vi "HFRR ADV v01.vi"() -> ()   [LabVIEW 2025] (continued)
                }
                frame 27 {
                  n3474 = property on="Boolean  4" class="Bool (strict)"("Boolean Text.Text"=w4454) -> ()  [unwired: 2 in, 2 out]
                }
                frame 28 {
                  n3475 = property on="Test \nStatus" class="Bool (strict)"("Boolean Text.Text"=w4455) -> ()  [unwired: 2 in, 2 out]
                }
                frame 29 {
                }
                frame 30 {
                }
                frame 31 {
                }
                frame 32 {
                  n3476 = property on="RSTCOF" class="Bool"("Boolean Text.Text"=w4457) -> ()  [unwired: 2 in, 2 out]
                  n3477 = property on="RST FF" class="Bool"("Boolean Text.Text"=w4457) -> ()  [unwired: 2 in, 2 out]
                  n3478 = property on="RST TEMP" class="Bool"("Boolean Text.Text"=w4457) -> ()  [unwired: 2 in, 2 out]
                  n3479 = property on="RSTV1 3" class="Bool"("Boolean Text.Text"=w4457) -> ()  [unwired: 2 in, 2 out]
                  n3480 = property on="rstv2" class="Bool"("Boolean Text.Text"=w4457) -> ()  [unwired: 2 in, 2 out]
                  n3481 = property on="RSTV1 2" class="Bool"("Boolean Text.Text"=w4457) -> ()  [unwired: 2 in, 2 out]
                  n3482 = property on="RST CP" class="Bool"("Boolean Text.Text"=w4457) -> ()  [unwired: 2 in, 2 out]
                }
                frame 33 {
                  "S 61" <- w4458
                }
                frame 34 {
                  "String 23" <- w4459
                }
                frame 35 {
                  n3483 = property on="Rh Before" class="DigNum (strict)"("Caption.Text"=w4460) -> ()  [unwired: 2 in, 2 out]
                }
                frame 36 {
                  n3484 = Match Pattern(string=w4461, regular expression=",") -> (before substring=→"bs":string, after substring=→"as":string)  [unwired: 1 in, 2 out]
                  n3485 = property on="Rh After" class="DigNum (strict)"("Caption.Text"=w4461) -> ()  [unwired: 2 in, 2 out]
                }
                frame 37 {
                  n3486 = Match Pattern(string=w4470, regular expression=",") -> (before substring=w4469:string, after substring=w4468:string)  [unwired: 1 in, 2 out]
                  "bs" <- w4469
                  "as" <- w4468
                  n3487 = Concatenate Strings(w4469, w4468) -> (w4465:string)
                  n3488 = property on="Humidity before test 2" class="DigNum (strict)"("Caption.Text"=w4465) -> ()  [unwired: 2 in, 2 out]
                  n3489 = Concatenate Strings(w4465, "=" ("string")) -> (w4466:string)
                  n3490 = local write "S 38"(w4466) -> ()
                }
                frame 38 {
                  n3491 = Match Pattern(string=w4477, regular expression=",") -> (before substring=w4476:string, after substring=w4475:string)  [unwired: 1 in, 2 out]
                  "bs" <- w4476
                  "as" <- w4475
                  n3492 = Concatenate Strings(w4476, w4475) -> (w4472:string)
                  n3493 = property on="Humidity after test 2" class="DigNum (strict)"("Caption.Text"=w4472) -> ()  [unwired: 2 in, 2 out]
                  n3494 = Concatenate Strings(w4472, "=" ("string")) -> (w4474:string)
                  n3495 = local write "S 39"(w4474) -> ()
                }
                frame 39 {
                  n3496 = Match Pattern(string=w4484, regular expression=",") -> (before substring=w4483:string, after substring=w4482:string)  [unwired: 1 in, 2 out]
                  "bs" <- w4483
                  "as" <- w4482
                  n3497 = Concatenate Strings(w4483, w4482) -> (w4479:string)
                  n3498 = property on="Temperature before test 2" class="DigNum (strict)"("Caption.Text"=w4479) -> ()  [unwired: 2 in, 2 out]
                  n3499 = Concatenate Strings(w4479, "=" ("string")) -> (→"String 34":string)
                }
                frame 40 {
                  n3500 = Match Pattern(string=w4491, regular expression=",") -> (before substring=w4490:string, after substring=w4489:string)  [unwired: 1 in, 2 out]
                  "bs" <- w4490
                  "as" <- w4489
                  n3501 = Concatenate Strings(w4490, w4489) -> (w4486:string)
                  n3502 = property on="Temperature after test 2" class="DigNum (strict)"("Caption.Text"=w4486) -> ()  [unwired: 2 in, 2 out]
                  n3503 = Concatenate Strings(w4486, "=" ("string")) -> (→"String 35":string)
                  n3504 = property on="Temperature after test" class="DigNum (strict)"("Caption.Text"=w4486) -> ()  [unwired: 2 in, 2 out]
                }
                frame 41 {
                  n3505 = property on="AVP 2" class="DigNum (strict)"("Caption.Text"=w4495) -> ()  [unwired: 2 in, 2 out]
                  n3506 = Concatenate Strings(w4495, "=" ("string")) -> (→"String 36":string)
                }
                frame 42 {
                  n3507 = property on="MWSD 2" class="DigNum (strict)"("Caption.Text"=w4498) -> ()  [unwired: 2 in, 2 out]
                  n3508 = Concatenate Strings(w4498, "=" ("string")) -> (→"String 37":string)
                }
                frame 43 {
                  n3509 = property on="HCF 2" class="DigNum (strict)"("Caption.Text"=w4501) -> ()  [unwired: 2 in, 2 out]
                  n3510 = Concatenate Strings(w4501, "=" ("string")) -> (→"String 38":string)
                }
                frame 44 {
                  n3511 = Concatenate Strings(w4503, "=" ("string")) -> (→"String 39":string)
                  n3512 = property on="WS1.4 2" class="DigNum (strict)"("Caption.Text"=w4503) -> ()  [unwired: 2 in, 2 out]
                }
                frame 45 {
                }
                frame 46 {
                  n3513 = local write "S 47"(w4506) -> ()
                }
                frame 47 {
                  n3514 = local write "S 48"(w4507) -> ()
                }
                frame 48 {
                  n3515 = local write "S 49"(w4508) -> ()
                }
                frame 49 {
                  n3516 = local write "S 50"(w4509) -> ()
                }
                frame 50 {
                  n3517 = local write "S 51"(w4510) -> ()
                }
                frame 51 {
                  n3518 = local write "S 52"(w4511) -> ()
                }
                frame 52 {
                  n3519 = local write "S 53"(w4512) -> ()
                }
                frame 53 {
                  n3520 = local write "S 54"(w4513) -> ()
                }
                frame 54 {
                  n3521 = local write "S 55"(w4514) -> ()
                }
                frame 55 {
                  n3522 = local write "S 56"(w4515) -> ()
                }
                frame 56 {
                  n3523 = local write "S 57"(w4516) -> ()
                }
                frame 57 {
                  n3524 = local write "S 58"(w4517) -> ()
                }
                frame 58 {
                  n3525 = local write "S 59"(w4518) -> ()
                }
                frame 59 {
                  n3526 = local write "S 60"(w4519) -> ()
                }
                frame 60 {
                  n3527 = local write "S 62"(w4520) -> ()
                }
                frame 61 {
                  n3528 = local write "S 63"(w4521) -> ()
                }
                frame 62 {
                  n3529 = local write "S 64"(w4522) -> ()
                }
                frame 63 {
                  n3530 = local write "S 65"(w4523) -> ()
                }
                frame 64 {
                  n3531 = local write "S 66"(w4524) -> ()
                }
                frame 65 {
                  n3532 = local write "S 67"(w4525) -> ()
                }
                frame 66 {
                  n3533 = local write "S 68"(w4526) -> ()
                }
                frame 67 {
                  n3534 = local write "S 69"(w4527) -> ()
                }
                frame 68 {
                  n3535 = local write "S 70"(w4528) -> ()
                }
                frame 69 {
                  n3536 = local write "S 71"(w4529) -> ()
                }
                frame 70 {
                  n3537 = local write "S 72"(w4530) -> ()
                }
                frame 71 {
                  n3538 = local write "S 73"(w4531) -> ()
                }
                frame 72 {
                  n3539 = local write "S 74"(w4532) -> ()
                }
                frame 73 {
                  n3540 = local write "S 75"(w4533) -> ()
                }
                frame 74 {
                  n3541 = local write "S 76"(w4534) -> ()
                }
                frame 75 {
                  n3542 = local write "S 77"(w4535) -> ()
                }
                frame 76 {
                  n3543 = local write "S 78"(w4536) -> ()
                }
                frame 77 {
                  n3544 = local write "S 79"(w4537) -> ()
                }
                frame 79 {
                  n3545 = property on="Sample Temperature ( °C )" class="XYGraph (strict)"("Y Scale.Name Label.Text"=w4538) -> ()  [unwired: 2 in, 2 out]
                }
                frame 80 {
                  n3546 = local write "S 81"(w4539) -> ()
                  n3547 = property on="Humidity ( %RH )" class="XYGraph (strict)"("Y Scale.Name Label.Text"=w4539) -> ()  [unwired: 2 in, 2 out]
                }
                frame 78 {
                  n3548 = property on="Air Temperature  ( °C )" class="XYGraph (strict)"("X Scale.Name Label.Text"=w4540) -> ()  [unwired: 2 in, 2 out]
                  n3549 = property on="Humidity ( %RH )" class="XYGraph (strict)"("X Scale.Name Label.Text"=w4540) -> ()  [unwired: 2 in, 2 out]
                  n3550 = property on="Sample Temperature ( °C )" class="XYGraph (strict)"("X Scale.Name Label.Text"=w4540) -> ()  [unwired: 2 in, 2 out]
                  n3551 = property on="Coefficient Of Friction" class="XYGraph (strict)"("X Scale.Name Label.Text"=w4540) -> ()  [unwired: 2 in, 2 out]
                }
                frame 81 {
                  n3552 = property on="Air Temperature  ( °C )" class="XYGraph (strict)"("Y Scale.Name Label.Text"=w4541) -> ()  [unwired: 2 in, 2 out]
                }
                frame 82 {
                  n3553 = local write "S 84"(w4542) -> ()
                }
                frame 83 {
                  n3554 = local write "S 85"(w4543) -> ()
                }
                frame 84 {
                  n3555 = local write "S 86"(w4544) -> ()
                }
                frame 85 {
                  n3556 = local write "S 87"(w4545) -> ()
                }
                frame 86 {
                  n3557 = local write "S 88"(w4546) -> ()
                }
                frame 87 {
                }
                frame 88 {
                  n3558 = local write "S 90"(w4548) -> ()
                }
                frame 89 {
                  n3559 = local write "S 91"(w4549) -> ()
                }
                frame 90 {
                  n3560 = local write "S 92"(w4550) -> ()
                }
                frame 91 {
                  n3561 = local write "S 93"(w4551) -> ()
                }
                frame 92 {
                  n3562 = local write "S 94"(w4552) -> ()
                }
                frame 93 {
                  n3563 = local write "S 95"(w4553) -> ()
                }
                frame 94 {
                  n3564 = local write "S 96"(w4554) -> ()
                }
                frame 95 {
                  n3565 = local write "S 97"(w4555) -> ()
                }
                frame 96 {
                  n3566 = local write "S 98"(w4556) -> ()
                }
                frame 97 {
                  n3567 = local write "S 99"(w4557) -> ()
                }
                frame 98 {
                  n3568 = local write "S 100"(w4558) -> ()
                }
                frame 99 {
                  n3569 = local write "S 101"(w4559) -> ()
                }
                frame 100 {
                  n3570 = local write "S 102"(w4560) -> ()
                }
                frame 101 {
                  n3571 = local write "S 103"(w4561) -> ()
                }
                frame 102 {
                  n3572 = local write "S 104"(w4562) -> ()
                }
                frame 103 {
                  n3573 = local write "S 105"(w4563) -> ()
                }
                frame 104 {
                  n3574 = local write "S 106"(w4564) -> ()
                }
                frame 105 {
                }
                frame 106 {
                  n3575 = property on="OK Button 17" class="Bool (strict)"("Boolean Text.Text"=w4565) -> ()  [unwired: 2 in, 2 out]
                }
                frame 107 {
                  n3576 = property on="OK Button 16" class="Bool (strict)"("Boolean Text.Text"=w4566) -> ()  [unwired: 2 in, 2 out]
                }
                frame 108 {
                  n3577 = property on="TITTLE" class="Str"("Caption.Text"=w4567) -> ()  [unwired: 2 in, 2 out]
                }
                frame 109 {
                  "String 30" <- w4568
                }
                frame 110 {
                  n3578 = property on="Test Date" class="Str"("Caption.Text"=w4569) -> ()  [unwired: 2 in, 2 out]
                  "String 31" <- w4569
                }
                frame 111 {
                  n3579 = property on="Sample ID" class="Str"("Caption.Text"=w4570) -> ()  [unwired: 2 in, 2 out]
                  "String 32" <- w4570
                }
                frame 112 {
                  n3580 = property on="Tested by" class="Str"("Caption.Text"=w4571) -> ()  [unwired: 2 in, 2 out]
                  "String 33" <- w4571
                }
                frame 113 {
                  n3581 = property on="System Configured Printers 2" class="Arr (strict)"("Caption.Text"=w4572) -> ()  [unwired: 2 in, 2 out]
                }
                frame 114 {
                  n3582 = property on="Selected Printer" class="Str"("Caption.Text"=w4573) -> ()  [unwired: 2 in, 2 out]
                }
                frame 115 {
                  n3583 = property on="Select Printer 3" class="DigNum (strict)"("Caption.Text"=w4574) -> ()  [unwired: 2 in, 2 out]
                }
                frame 116 {
                  n3584 = property on="Print" class="Bool (strict)"("Boolean Text.Text"=w4575) -> ()  [unwired: 2 in, 2 out]
                }
                frame 117 {
                  "String 41" <- w4576
                }
                frame 118 {
                  n3585 = property on="tested by" class="Str"("Caption.Text"=w4577) -> ()  [unwired: 2 in, 2 out]
                }
                frame 119 {
                }
                frame 120 {
                  n3586 = property on="Export" class="Bool (strict)"("Boolean Text.Text"=w4578) -> ()  [unwired: 2 in, 2 out]
                }
                frame 121 {
                }
                frame 122 {
                }
                frame 123 {
                  n3587 = property on="Select File Type" class="Enum (strict)"("Caption.Text"=w4581) -> ()  [unwired: 2 in, 2 out]
                }
                frame 124 {
                  n3588 = property on="s.NO" class="Str"("Caption.Text"=w4582) -> ()  [unwired: 2 in, 2 out]
                  "String 45" <- w4582
                }
                frame 125 {
                  n3589 = property on="trip1 8" class="Bool (strict)"("Boolean Text.Text"=w4583) -> ()  [unwired: 2 in, 2 out]
                }
                frame 126, Default {
                }
              }
            }
          }
          frame #1 {
            w4591 = TRUE ("Visible")
            n3590 = local read "S 91"() -> (w4608:string)
            n3591 = local read "S 90"() -> (w4607:string)
            n3592 = local read "S 88"() -> (w4606:string)
            n3593 = property on="File Path" class="Path"("Caption.Text"=w4607) -> ()  [unwired: 2 in, 2 out]
            n3594 = local read "S 71"() -> (w4601:string)
            n3595 = local read "S 86"() -> (w4603:string)
            n3596 = local read "S 85"() -> (w4604:string)
            n3597 = local read "S 87"() -> (w4602:string)
            n3598 = local read "S 84"() -> (w4605:string)
            n3599 = local read "S 103"() -> (w4590:string)
            n3600 = local read "S 104"() -> (w4589:string)
            n3601 = property on="Password" class="Str"("Caption.Text"=w4604) -> ()  [unwired: 2 in, 2 out]
            n3602 = property on="EDIT" class="Bool (strict)"("Boolean Text.Text"=w4601) -> ()  [unwired: 2 in, 2 out]
            n3603 = property on="SAVE" class="Bool (strict)"("Boolean Text.Text"=w4605) -> ()  [unwired: 2 in, 2 out]
            n3604 = Build Array(w4590, w4589) -> (w4588:string[])
            n3605 = property on="Heater Button" class="Bool (strict)"("Strings [4]"=w4588) -> ()  [unwired: 2 in, 2 out]
            n3606 = local read "S 92"() -> (w4600:string)
            n3607 = local read "S 93"() -> (w4599:string)
            n3608 = local read "S 105"() -> (w4586:string)
            n3609 = local read "S 106"() -> (w4585:string)
            n3610 = Build Array(w4600, w4599) -> ()  [unwired: 1 out]
            n3611 = Build Array(w4586, w4585) -> (w4587:string[])
            n3612 = local read "S 95"() -> (w4597:string)
            n3613 = local read "S 94"() -> (w4598:string)
            n3614 = local read "bs"() -> (w4613:string)
            n3615 = local read "as"() -> (w4614:string)
            n3616 = property on="Humidity" class="Bool (strict)"("Strings [4]"=w4587) -> ()  [unwired: 2 in, 2 out]
            n3617 = Concatenate Strings(w4613, "\r", w4614) -> ()  [unwired: 1 out]
            n3618 = property on="Rh After" class="DigNum (strict)"("Caption.Size to Text?"=TRUE ("Caption.Size to Text")) -> ()  [unwired: 2 in, 2 out]
            n3619 = local read "S 48"() -> (w4637:string)
            n3620 = local read "S 50"() -> (w4635:string)
            n3621 = local read "S 51"() -> (w4634:string)
            n3622 = local read "S 49"() -> (w4636:string)
            n3623 = local read "S 52"() -> (w4633:string)
            n3624 = local read "as"() -> (w4618:string)
            n3625 = local read "bs"() -> (w4619:string)
            n3626 = local read "S 56"() -> (w4632:string)
            n3627 = local read "S 57"() -> (w4631:string)
            n3628 = local read "S 58"() -> (w4630:string)
            n3629 = local read "S 59"() -> (w4629:string)
            n3630 = property on="OPEN" class="Bool (strict)"("Boolean Text.Text"=w4633) -> ()  [unwired: 2 in, 2 out]
            n3631 = property on="OPEN 1" class="Bool (strict)"("Boolean Text.Text"=w4637) -> ()  [unwired: 2 in, 2 out]
            n3632 = property on="OPEN 2" class="Bool (strict)"("Boolean Text.Text"=w4636) -> ()  [unwired: 2 in, 2 out]
            n3633 = property on="OPEN 3" class="Bool (strict)"("Boolean Text.Text"=w4635) -> ()  [unwired: 2 in, 2 out]
            n3634 = property on="OPEN 4" class="Bool (strict)"("Boolean Text.Text"=w4634) -> ()  [unwired: 2 in, 2 out]
            n3635 = Concatenate Strings(w4619, "\r", w4618) -> ()  [unwired: 1 out]
            n3636 = local read "S 102"() -> (w4592:string)
            n3637 = property on="КОФ1" class="DigNum (strict)"("Caption.Text"=w4632) -> ()  [unwired: 2 in, 2 out]
            n3638 = local read "S 98"() -> (w4596:string)
            n3639 = local read "S 99"() -> (w4595:string)
            n3640 = local read "S 100"() -> (w4594:string)
            n3641 = local read "S 101"() -> (w4593:string)
            n3642 = property on="КОФ2" class="DigNum (strict)"("Caption.Text"=w4631) -> ()  [unwired: 2 in, 2 out]
            n3643 = property on="КОФ3" class="DigNum (strict)"("Caption.Text"=w4630) -> ()  [unwired: 2 in, 2 out]
            n3644 = property on="КОФ4" class="DigNum (strict)"("Caption.Text"=w4629) -> ()  [unwired: 2 in, 2 out]
            n3645 = local read "bs"() -> (w4617:string)
            n3646 = local read "as"() -> (w4616:string)
            n3647 = local read "S 60"() -> (w4628:string)
            n3648 = local read "S 54"() -> (w4638:string)
            n3649 = Concatenate Strings(w4617, "\r", w4616) -> ()  [unwired: 1 out]
            n3650 = Concatenate Strings(w4638, w4628) -> ()  [unwired: 1 out]
            n3651 = local read "S 77"() -> (→"String 43":string)
            n3652 = local read "S 76"() -> (w4611:string)
            n3653 = local read "S 78"() -> (w4610:string)
            n3654 = local read "S 71"() -> (w4622:string)
            n3655 = local read "S 66"() -> (w4627:string)
            n3656 = local read "S 67"() -> (w4626:string)
            n3657 = local read "S 68"() -> (w4625:string)
            n3658 = local read "S 69"() -> (w4624:string)
            n3659 = local read "S 70"() -> (w4623:string)
            n3660 = property on="AIR TEMP" class="DigNum (strict)"("Caption.Text"=w4610) -> ()  [unwired: 2 in, 2 out]
            n3661 = property on="Set Strk" class="DigNum (strict)"("Caption.Text"=w4611) -> ()  [unwired: 2 in, 2 out]
            n3662 = property on="SPEED OUT:" class="DigNum (strict)"("Caption.Text"=w4625) -> ()  [unwired: 2 in, 2 out]
            n3663 = property on="EDIT" class="Bool (strict)"("Boolean Text.Text"=w4622) -> ()  [unwired: 2 in, 2 out]
            n3664 = local read "S 79"() -> (w4609:string)
          }
          frame #2 {
          }
        }
        n3665 = local write "Lan flag"(10.0 ("Lan flag")) -> ()
      }
      frame Enabled {
      }
    }
    n3666 = Wait (ms)(milliseconds to wait=u32 2000) -> ()  [unwired: 1 out]
    n3667 = local read "Quit"() -> (w4412:bool)
  }
  n3668 = while {
    shift-right: [w4644] -> _
    shift-left: _ -> [w4645]
    shift-right: [w4642] -> _
    shift-left: T19 {"Read Heave and Surge"="", "Bytes at Heave Port"=0.0, "Heave and Surge COM Port:"="COM9", "Com Port 2"="COM7", "Residual Due"="", "Heave COM Status 2"=TRUE, "Heave COM Status"=TRUE, "Port 2"=TRUE, "Sway PPR"=6400.0, "Surge PPR"=6400.0, "Heave PPR"=6400.0, "Sway Pitch"=2.0, "Surge Pitch"=3.0, "Heave Pitch"=4.0, "Sway Pulses/mm"=320.0, "Surge Pulses/mm"=1600.0, "Heave Pulses/mm"=1600.0, "inner loop"=0.0, "Read Heave and Surge 2"="", "String 36"="", "Write S"=FALSE, "WriteCC1"=[""], "Heave COM Loop"=0, "LastCom"="", "EXIT"=FALSE, "Error Heave"={"status"=TRUE, "code"=-1073807343, "source"=""}} -> [w4641]
    shift-right: [w4639] -> _
    shift-left: enum16{"init", "MAIN", "Panel Close"}."init" -> [w4640]
    stop <- w4643 stop-if-true
    # "HUMIDITY LOOP LOGIC"
    n3669 = case shown="\"MAIN\"" w4640 {
      tunnel: w4645 -> [w4659 w4684 w4783 w4785]
      tunnel: [w4654 w4668 w4783 w4785] -> w4644
      tunnel: [_ _ TRUE _] -> w4643
      tunnel: [w4651 w4669 w4781 w4784] -> w4642
      tunnel: w4641 -> [w4656 w4683 w4781 w4784]
      tunnel: [enum16{"init", "MAIN", "Panel Close"}."MAIN" w4678 _ _] -> w4639
      frame "init" {
        n3670 = local read "C3 :"() -> (w4646:refnum<visa-resource-name>)
        n3671 = Bundle By Name(cluster=w4656, "Heave and Surge COM Port:"=w4646) -> (w4655:T19)
        n3672 = call "Instrument fgv uno.vi"("Enum"=T32."INIT", "error in (no error) 2"=w4659, "INPUT"=w4655) -> ("error"=w4657:errorcluster, "output"=w4653:T19)  [unwired: 6 in, 1 out]
        n3673 = case shown="Error" w4657 {
          selector: w4657 -> [w4661 _]
          tunnel: [w4661 w4665] -> w4654
          tunnel: w4653 -> [w4660 w4663]
          tunnel: [w4660 w4662] -> w4652
          frame No Error {
          }
          frame Error {
            n3674 = call "Instrument fgv uno.vi"("Enum"=T32."ERROR INIT", "INPUT"=w4663) -> ("error"=w4666:errorcluster, "output"=w4662:T19)  [unwired: 7 in, 1 out]
            n3675 = call <vilib>:"Clear Errors.vi"("error in (no error)"=w4666) -> ("error out"=w4665:errorcluster)  [unwired: 5 in, 1 out]
          }
        }
        n3676 = local read "LastCom Humidity"() -> (w4649:string)
        n3677 = Unbundle By Name(w4652) -> ("Heave COM Status 2"=→"COM Status":bool, "Error Heave"=→"Error":errorcluster)  [unwired: 1 out]
        n3678 = Bundle By Name(cluster=w4652, "LastCom"=w4649) -> (w4651:T19)
      }
      frame "MAIN" {
        n3679 = Unbundle By Name(w4683) -> ("Com Port 2"=w4673:refnum<visa-resource-name>)
        n3680 = local read "C3 :"() -> (w4674:refnum<visa-resource-name>)
        n3681 = local write "COM Port Humidity :"(w4673) -> ()
        n3682 = Bundle By Name(cluster=w4683, "Heave and Surge COM Port:"=w4674) -> (w4682:T19)
        n3683 = Equal?(x=w4673, y=w4674) -> (x = y?=w4687:bool)
        n3684 = case shown="True" w4687 {
          tunnel: [w4727 w4745] -> w4672
          tunnel: w4684 -> [w4728 w4751]
          tunnel: w4682 -> [w4726 w4749]
          tunnel: [w4725 w4744] -> w4671
          frame False {
            n3685 = call <vilib>:"Clear Errors.vi"("error in (no error)"=w4728) -> ("error out"=w4724:errorcluster)  [unwired: 5 in, 1 out]
            n3686 = call "Instrument fgv uno.vi"("Enum"=T32."ERROR INIT", "error in (no error) 2"=w4724, "INPUT"=w4726) -> ("error"=w4730:errorcluster, "output"=w4725:T19)  [unwired: 6 in, 1 out]
            n3687 = call <vilib>:"Clear Errors.vi"("error in (no error)"=w4730) -> ("error out"=w4727:errorcluster)  [unwired: 5 in, 1 out]
          }
          frame True {
            n3688 = call "Instrument fgv uno.vi"("Enum"=T32."READ", "error in (no error) 2"=w4751, "milliseconds to wait"="milliseconds to wait 2", "INPUT"=w4749) -> ("error"=w4750:errorcluster, "output"=w4743:T19)  [unwired: 5 in, 1 out]
            n3689 = Bundle By Name(cluster=w4743, "String 36"="WRITE HUMIDITY") -> (w4742:T19)
            n3690 = case shown="True" "Write Humidity" {
              selector: "Write Humidity" -> [_ w4780]
              tunnel: w4750 -> [w4773 w4779]
              tunnel: [w4773 w4778] -> w4740
              tunnel: w4742 -> [w4772 w4776]
              tunnel: [w4772 w4775] -> w4739
              frame False {
              }
              frame True {
                n3691 = Not(x=w4780) -> (.not. x?=w4774:bool)
                n3692 = local write "Write Humidity"(w4774) -> ()
                n3693 = call "Instrument fgv uno.vi"("Enum"=T32."MANUAL WRITE", "error in (no error) 2"=w4779, "INPUT"=w4776) -> ("error"=w4778:errorcluster, "output"=w4775:T19)  [unwired: 6 in, 1 out]
              }
            }
            n3694 = Array Size(array="WriteHumidity") -> (size(s)=w4737:i32)
            n3695 = Greater Than 0?(x=w4737) -> (x > 0?=w4736:bool)
            n3696 = call "Instrument fgv uno.vi"("Enum"=T32."WRITE", "error in (no error) 2"=w4740, "WriteCC1"="WriteHumidity", "INPUT"=w4739) -> ("error"=w4747:errorcluster, "WriteCC1 2"=w4738:string[], "output"=w4746:T19)  [unwired: 5 in]
            n3697 = case shown="Error" w4747 {
              selector: w4747 -> [w4754 w4759]
              tunnel: w4746 -> [w4755 w4763]
              tunnel: [w4755 w4762] -> w4744
              tunnel: [w4754 w4760] -> w4745
              frame No Error {
              }
              frame Error {
                n3698 = Unbundle By Name(w4759) -> ("code"=w4758:i32)
                n3699 = Equal?(x=w4758, y=56) -> (x = y?=w4756:bool)
                n3700 = case shown="True" w4756 {
                  tunnel: w4763 -> [w4769 w4770]
                  tunnel: [w4768 w4770] -> w4762
                  tunnel: [w4767 w4771] -> w4761
                  tunnel: w4759 -> [w4764 w4771]
                  frame False {
                    n3701 = call <vilib>:"Clear Errors.vi"("error in (no error)"=w4764) -> ("error out"=w4765:errorcluster)  [unwired: 5 in, 1 out]
                    n3702 = call "Instrument fgv uno.vi"("Enum"=T32."ERROR INIT", "error in (no error) 2"=w4765, "INPUT"=w4769) -> ("error"=w4767:errorcluster, "output"=w4768:T19)  [unwired: 6 in, 1 out]
                  }
                  frame True {
                  }
                }
                n3703 = call <vilib>:"Clear Errors.vi"("error in (no error)"=w4761) -> ("error out"=w4760:errorcluster)  [unwired: 5 in, 1 out]
              }
            }
            n3704 = case shown="True" w4736 {
              tunnel: w4738 -> [_ w4753]
              frame False {
              }
              frame True {
                n3705 = local write "WriteHumidity"(w4753) -> ()
              }
            }
            n3706 = Unbundle By Name(w4744) -> ("LastCom"=→"LastCom Humidity":string, "Read Heave and Surge"=→"Read HUMIDITY":string)
          }
        }
        n3707 = Unbundle By Name(w4671) -> ("Heave COM Status 2"=w4686:bool, "Error Heave"=w4675:errorcluster, "Bytes at Heave Port"=→"Bytes at Humidity Port  2":dbl)  [unwired: 1 out]
        n3708 = Unbundle By Name(w4675) -> ("status"=→"Humidity Port":bool)
        n3709 = Not(x=w4686) -> (.not. x?=w4676:bool)
        n3710 = local write "Error"(w4675) -> ()
        n3711 = local read "Quit"() -> (w4679:bool)
        n3712 = local write "COM Status"(w4676) -> ()
        n3713 = Select(t=enum16{"init", "MAIN", "Panel Close"}."Panel Close", s=w4679, f=enum16{"init", "MAIN", "Panel Close"}."MAIN") -> (s? t:f=w4678:enum16{"init", "MAIN", "Panel Close"})
        n3714 = disable-structure shown="Enabled" {
          disable-tunnel: w4672 -> [w4692 w4704]
          disable-tunnel: w4671 -> [w4691 w4705]
          disable-tunnel: [w4689 w4705] -> w4670
          disable-tunnel: [w4688 w4704] -> w4667
          frame Disabled {
            n3715 = local read "Humidity 2"() -> (w4690:bool)
            n3716 = case shown="True" w4690 {
              selector: w4690 -> [_ w4695]
              tunnel: w4692 -> [w4693 w4700]
              tunnel: [w4693 w4699] -> w4688
              tunnel: w4691 -> [w4694 w4698]
              tunnel: [w4694 w4697] -> w4689
              frame False {
              }
              frame True {
                n3717 = Not(x=w4695) -> (.not. x?=→"Humidity 2":bool)
                n3718 = call <vilib>:"Clear Errors.vi"("error in (no error)"=w4700) -> ("error out"=w4703:errorcluster)  [unwired: 5 in, 1 out]
                n3719 = call "Instrument fgv uno.vi"("Enum"=T32."ERROR INIT", "error in (no error) 2"=w4703, "INPUT"=w4698) -> ("error"=w4701:errorcluster, "output"=w4697:T19)  [unwired: 6 in, 1 out]
                n3720 = call <vilib>:"Clear Errors.vi"("error in (no error)"=w4701) -> ("error out"=w4699:errorcluster)  [unwired: 5 in, 1 out]
              }
            }
          }
          frame Enabled {
          }
        }
        n3721 = case shown="Error .." w4667 {
          tunnel: w4670 -> [w4710 w4722]
          tunnel: w4667 -> [w4709 w4723]
          tunnel: [w4708 w4722] -> w4669
          tunnel: [w4707 w4723] -> w4668
          frame No Error {
            n3722 = First Call?() -> (First Call?: T/F=w4706:bool)
            n3723 = case shown="True" w4706 {
              tunnel: w4709 -> [w4711 w4718]
              tunnel: [w4711 w4717] -> w4707
              tunnel: w4710 -> [w4712 w4716]
              tunnel: [w4712 w4715] -> w4708
              frame False {
              }
              frame True {
                n3724 = call "Stall Data Flow.vim"("value in"=w4718, "milliseconds to wait"=u32 1000) -> ("value out"=w4714:errorcluster)  [unwired: 1 out]
                n3725 = call <vilib>:"Clear Errors.vi"("error in (no error)"=w4714) -> ("error out"=w4721:errorcluster)  [unwired: 5 in, 1 out]
                n3726 = call "Instrument fgv uno.vi"("Enum"=T32."ERROR INIT", "error in (no error) 2"=w4721, "INPUT"=w4716) -> ("error"=w4719:errorcluster, "output"=w4715:T19)  [unwired: 6 in, 1 out]
                n3727 = call <vilib>:"Clear Errors.vi"("error in (no error)"=w4719) -> ("error out"=w4717:errorcluster)  [unwired: 5 in, 1 out]
              }
            }
          }
          frame Error {
          }
        }
      }
      frame "Panel Close" {
      }
      frame Default {
      }
    }
  }
  n3728 = while {
    shift-right: [w4786] -> _
    shift-left: DEMO_Main_Enum."INIT" -> [w4787]
    stop <- w4788 stop-if-true
    # "DEMO MODE"
    n3729 = case shown="\"DEMO STOP\"" w4787 {
      tunnel: [w4789 w4793 w4818 w4822 w4848 w5030 w5074 DEMO_Main_Enum."INIT"] -> w4786
      frame "INIT", Default {
        n3730 = property on="DEMO" class="Bool (strict)"() -> ("Value"=w4792:bool)  [unwired: 2 in, 2 out]
        n3731 = Select(t=DEMO_Main_Enum."DEMO START", s=w4792, f=DEMO_Main_Enum."INIT") -> (s? t:f=w4789:T18)
      }
      frame "DEMO START" {
        n3732 = stacked-sequence {
          tunnel: [_ w4798] -> w4793
          frame #0 {
            w4794 = "" ("USERNAME")
            n3733 = local write "USERNAME"(w4794) -> ()
            n3734 = local write "USER ID"(w4794) -> ()
            n3735 = local write "Main Dashboard Buttons"(T1."Home" ("Main Dashboard Buttons")) -> ()
            n3736 = local write "main tab sub"(enum32{"Page 1", "Page 2"}."Page 1" ("main tab sub")) -> ()
            n3737 = local write "Main Tab"(T4."HOME" ("Main Tab")) -> ()
          }
          frame #1 {
            w4804 = u32 800 ("milliseconds to wait")
            n3738 = property on="USERNAME" class="Str"("Value"="ADMIN" ("USERNAME")) -> (error out=w4815:errorcluster)  [unwired: 2 in, 1 out]
            n3739 = call "Stall Data Flow.vim"("value in"=w4815, "milliseconds to wait"=w4804) -> ("value out"=w4814:errorcluster)  [unwired: 1 out]
            n3740 = property on="USER ID" class="Str"(error in=w4814, "Value"="001" ("USER ID")) -> (error out=w4812:errorcluster)  [unwired: 1 in, 1 out]
            n3741 = call "Stall Data Flow.vim"("value in"=w4812, "milliseconds to wait"=w4804) -> ("value out"=w4811:errorcluster)  [unwired: 1 out]
            n3742 = property on="Main Tab" class="TabCtl (strict)"(error in=w4811, "Value"=T4."Test Setup" ("Main Tab")) -> (error out=w4809:errorcluster)  [unwired: 1 in, 1 out]
            n3743 = call "Stall Data Flow.vim"("value in"=w4809, "milliseconds to wait"=w4804) -> ("value out"=w4807:errorcluster)  [unwired: 1 out]
            n3744 = property on="main tab sub" class="TabCtl (strict)"(error in=w4807, "Value"=enum32{"Page 1", "Page 2"}."Page 2" ("main tab sub")) -> (error out=w4806:errorcluster)  [unwired: 1 in, 1 out]
            n3745 = call "Stall Data Flow.vim"("value in"=w4806, "milliseconds to wait"=w4804) -> ("value out"=w4805:errorcluster)  [unwired: 1 out]
            n3746 = property on="Main Dashboard Buttons" class="RadioBtnsControl (strict)"(error in=w4805, "Value"=T1."Test Setup" ("Main Dashboard Buttons")) -> ()  [unwired: 1 in, 2 out]
            n3747 = property on="DEMO" class="Bool (strict)"() -> ("Value"=w4802:bool)  [unwired: 2 in, 2 out]
            n3748 = Not(x=w4802) -> (.not. x?=w4801:bool)
            n3749 = Select(t=DEMO_Main_Enum."DEMO STOP", s=w4801, f=DEMO_Main_Enum."MAIN SCREEN  ENTRY") -> (s? t:f=w4798:T18)
          }
        }
      }
      frame "MAIN SCREEN  ENTRY" {
        n3750 = property on="DEMO" class="Bool (strict)"() -> ("Value"=w4821:bool)  [unwired: 2 in, 2 out]
        n3751 = Not(x=w4821) -> (.not. x?=w4820:bool)
        n3752 = Select(t=DEMO_Main_Enum."DEMO STOP", s=w4820, f=DEMO_Main_Enum."TEST PARAMETERS") -> (s? t:f=w4818:T18)
      }
      frame "TEST PARAMETERS" {
        n3753 = stacked-sequence {
          tunnel: [_ DEMO_Main_Enum."DASHBOARD"] -> w4823
          frame #0 {
            w4827 = u32 800 ("milliseconds to wait")
            n3754 = property on="FILE" class="Str"("Value"="DEMO TEST" ("FILE")) -> (error out=w4845:errorcluster)  [unwired: 2 in, 1 out]
            n3755 = call "Stall Data Flow.vim"("value in"=w4845, "milliseconds to wait"=w4827) -> ("value out"=w4843:errorcluster)  [unwired: 1 out]
            n3756 = property on="Batch Ref Num :" class="Str"(error in=w4843, "Value"="DEMO SAMPLE" ("Batch Ref Num :")) -> (error out=w4842:errorcluster)  [unwired: 1 in, 1 out]
            n3757 = call "Stall Data Flow.vim"("value in"=w4842, "milliseconds to wait"=w4827) -> ("value out"=w4841:errorcluster)  [unwired: 1 out]
            n3758 = property on="Fuel Discription :" class="Str"(error in=w4841, "Value"="DEMO FUEL" ("Fuel Discription :")) -> (error out=w4839:errorcluster)  [unwired: 1 in, 1 out]
            n3759 = call "Stall Data Flow.vim"("value in"=w4839, "milliseconds to wait"=w4827) -> ("value out"=w4837:errorcluster)  [unwired: 1 out]
            n3760 = property on="Remarks :" class="Str"(error in=w4837, "Value"="DEMO TEST" ("Remarks :")) -> (error out=w4836:errorcluster)  [unwired: 1 in, 1 out]
            n3761 = call "Stall Data Flow.vim"("value in"=w4836, "milliseconds to wait"=w4827) -> ("value out"=w4834:errorcluster)  [unwired: 1 out]
            n3762 = property on="TEST STANDARD" class="Enum (strict)"(error in=w4834, "Value"=T5."ISO 12156" ("TEST STANDARD")) -> (error out=w4833:errorcluster)  [unwired: 1 in, 1 out]
            n3763 = call "Stall Data Flow.vim"("value in"=w4833, "milliseconds to wait"=w4827) -> ("value out"=w4832:errorcluster)  [unwired: 1 out]
            n3764 = property on="Main Tab" class="TabCtl (strict)"(error in=w4832, "Value"=T4."Acquire" ("Main Tab")) -> (error out=w4830:errorcluster)  [unwired: 1 in, 1 out]
            n3765 = call "Stall Data Flow.vim"("value in"=w4830, "milliseconds to wait"=w4827) -> ("value out"=w4828:errorcluster)  [unwired: 1 out]
            n3766 = property on="Main Dashboard Buttons" class="RadioBtnsControl (strict)"(error in=w4828, "Value"=T1."Dashboard" ("Main Dashboard Buttons")) -> ()  [unwired: 1 in, 2 out]
          }
          frame #1 {
          }
        }
        n3767 = property on="DEMO" class="Bool (strict)"() -> ("Value"=w4826:bool)  [unwired: 2 in, 2 out]
        n3768 = Not(x=w4826) -> (.not. x?=w4825:bool)
        n3769 = Select(t=DEMO_Main_Enum."DEMO STOP", s=w4825, f=w4823) -> (s? t:f=w4822:T18)
      }
      frame "DASHBOARD" {
        n3770 = stacked-sequence {
          tunnel: [_ _ DEMO_Main_Enum."IMAGING"] -> w4849
          frame #0 {
            n3771 = stacked-sequence {
              frame #0 {
                n3772 = local write "Main Dashboard Buttons"(T1."Dashboard" ("Main Dashboard Buttons")) -> ()
                n3773 = local write "Main Tab"(T4."Acquire" ("Main Tab")) -> ()
              }
              frame #1 {
                n3774 = local write "EVENT LOG"("" ("EVENT LOG")) -> ()
              }
              frame #2 {
                n3775 = Wait (ms)(milliseconds to wait=u32 50) -> ()  [unwired: 1 out]
              }
              frame #3 {
                n3776 = local read "EVENT LOG"() -> (w4861:string)
                n3777 = local read "FILE"() -> (w4857:string)
                n3778 = Concatenate Strings("File Name :" ("Content"), w4857) -> (w4858:string)
                n3779 = call "Event Log.vi"("Content"=w4858, "EVENT LOG"=w4861) -> ("EVENT LOG"=w4860:string)  [unwired: 8 in, 1 out]
                n3780 = local write "EVENT LOG"(w4860) -> ()
              }
              frame #4 {
                n3781 = Wait (ms)(milliseconds to wait=u32 50) -> ()  [unwired: 1 out]
              }
              frame #5 {
                n3782 = local read "Batch Ref Num :"() -> (w4863:string)
                n3783 = local read "EVENT LOG"() -> (w4867:string)
                n3784 = Concatenate Strings("Batch Ref No :" ("Content"), w4863) -> (w4864:string)
                n3785 = call "Event Log.vi"("Content"=w4864, "EVENT LOG"=w4867) -> ("EVENT LOG"=w4866:string)  [unwired: 8 in, 1 out]
                n3786 = local write "EVENT LOG"(w4866) -> ()
              }
              frame #6 {
                n3787 = Wait (ms)(milliseconds to wait=u32 50) -> ()  [unwired: 1 out]
              }
              frame #7 {
                n3788 = local read "EVENT LOG"() -> (w4873:string)
                n3789 = local read "tested by"() -> (w4869:string)
                n3790 = Concatenate Strings("Tested By :" ("Content"), w4869) -> (w4870:string)
                n3791 = call "Event Log.vi"("Content"=w4870, "EVENT LOG"=w4873) -> ("EVENT LOG"=w4872:string)  [unwired: 8 in, 1 out]
                n3792 = local write "EVENT LOG"(w4872) -> ()
              }
              frame #8 {
                n3793 = Wait (ms)(milliseconds to wait=u32 50) -> ()  [unwired: 1 out]
              }
              frame #9 {
                n3794 = local read "EVENT LOG"() -> (w4880:string)
                n3795 = local read "TEST STANDARD"() -> (w4876:T5)
                n3796 = case shown="\"CEC F-096-A-06\"" w4876 {
                  tunnel: ["ASTM D6079" "ISO 12156" "CEC F-096-A-06" "Custom"] -> w4875
                  frame "ASTM D6079", Default {
                  }
                  frame "ISO 12156" {
                  }
                  frame "CEC F-096-A-06" {
                  }
                  frame "Custom" {
                  }
                }
                n3797 = Concatenate Strings("Test Standard :" ("Content"), w4875) -> (w4877:string)
                n3798 = call "Event Log.vi"("Content"=w4877, "EVENT LOG"=w4880) -> ("EVENT LOG"=w4879:string)  [unwired: 8 in, 1 out]
                n3799 = local write "EVENT LOG"(w4879) -> ()
              }
              frame #10 {
                n3800 = Wait (ms)(milliseconds to wait=u32 50) -> ()  [unwired: 1 out]
              }
              frame #11 {
                n3801 = local read "Fuel Discription :"() -> (w4886:string)
                n3802 = Concatenate Strings("Fuel Description :" ("Content"), w4886) -> (w4887:string)
                n3803 = local read "EVENT LOG"() -> (w4890:string)
                n3804 = call "Event Log.vi"("Content"=w4887, "EVENT LOG"=w4890) -> ("EVENT LOG"=w4889:string)  [unwired: 8 in, 1 out]
                n3805 = local write "EVENT LOG"(w4889) -> ()
              }
              frame #12 {
                n3806 = Wait (ms)(milliseconds to wait=u32 50) -> ()  [unwired: 1 out]
              }
              frame #13 {
                n3807 = local read "EVENT LOG"() -> (w4896:string)
                n3808 = local read "Remarks :"() -> (w4892:string)
                n3809 = Concatenate Strings("Remarks :" ("Content"), w4892) -> (w4893:string)
                n3810 = call "Event Log.vi"("Content"=w4893, "EVENT LOG"=w4896) -> ("EVENT LOG"=w4895:string)  [unwired: 8 in, 1 out]
                n3811 = local write "EVENT LOG"(w4895) -> ()
              }
              frame #14 {
                n3812 = Wait (ms)(milliseconds to wait=u32 50) -> ()  [unwired: 1 out]
              }
              frame #15 {
                n3813 = local read "EVENT LOG"() -> (w4902:string)
                n3814 = local read "USER ID"() -> (w4898:string)
                n3815 = Concatenate Strings("Operator ID :" ("Content"), w4898) -> (w4900:string)
                n3816 = call "Event Log.vi"("Content"=w4900, "EVENT LOG"=w4902) -> ("EVENT LOG"=w4901:string)  [unwired: 8 in, 1 out]
                n3817 = local write "EVENT LOG"(w4901) -> ()
              }
              frame #16 {
                n3818 = Wait (ms)(milliseconds to wait=u32 50) -> ()  [unwired: 1 out]
              }
              frame #17 {
                n3819 = local read "EVENT LOG"() -> (w4910:string)
                n3820 = local read "Set Hz"() -> (w4906:dbl)
                n3821 = Number To Fractional String(number=w4906, precision (6)=i16 2) -> (F-format string=w4905:string)  [unwired: 2 in]
                n3822 = Concatenate Strings("Set Frequency [Hz] :" ("Content"), w4905) -> (w4908:string)
                n3823 = call "Event Log.vi"("Content"=w4908, "EVENT LOG"=w4910) -> ("EVENT LOG"=w4909:string)  [unwired: 8 in, 1 out]
                n3824 = local write "EVENT LOG"(w4909) -> ()
              }
              frame #18 {
                n3825 = Wait (ms)(milliseconds to wait=u32 50) -> ()  [unwired: 1 out]
              }
              frame #19 {
                n3826 = local read "EVENT LOG"() -> (w4918:string)
                n3827 = local read "NORMAL LOAD"() -> (w4913:dbl)
                n3828 = Number To Fractional String(number=w4913, precision (6)=i16 2) -> (F-format string=w4914:string)  [unwired: 2 in]
                n3829 = Concatenate Strings("Applied Load [grams] :" ("Content"), w4914) -> (w4916:string)
                n3830 = call "Event Log.vi"("Content"=w4916, "EVENT LOG"=w4918) -> ("EVENT LOG"=w4917:string)  [unwired: 8 in, 1 out]
                n3831 = local write "EVENT LOG"(w4917) -> ()
              }
              frame #20 {
                n3832 = Wait (ms)(milliseconds to wait=u32 50) -> ()  [unwired: 1 out]
              }
              frame #21 {
                n3833 = local read "EVENT LOG"() -> (w4926:string)
                n3834 = local read "Set Strk"() -> (w4921:dbl)
                n3835 = Number To Fractional String(number=w4921, precision (6)=i16 2) -> (F-format string=w4922:string)  [unwired: 2 in]
                n3836 = Concatenate Strings("Set Stroke [mm] :" ("Content"), w4922) -> (w4924:string)
                n3837 = call "Event Log.vi"("Content"=w4924, "EVENT LOG"=w4926) -> ("EVENT LOG"=w4925:string)  [unwired: 8 in, 1 out]
                n3838 = local write "EVENT LOG"(w4925) -> ()
              }
              frame #22 {
                n3839 = Wait (ms)(milliseconds to wait=u32 50) -> ()  [unwired: 1 out]
              }
              frame #23 {
                n3840 = local read "EVENT LOG"() -> (w4934:string)
                n3841 = local read "Set Temp"() -> (w4929:dbl)
                n3842 = Number To Fractional String(number=w4929, precision (6)=i16 2) -> (F-format string=w4930:string)  [unwired: 2 in]
                n3843 = Concatenate Strings("Set Temperature [deg C] :" ("Content"), w4930) -> (w4932:string)
                n3844 = call "Event Log.vi"("Content"=w4932, "EVENT LOG"=w4934) -> ("EVENT LOG"=w4933:string)  [unwired: 8 in, 1 out]
                n3845 = local write "EVENT LOG"(w4933) -> ()
              }
              frame #24 {
                n3846 = Wait (ms)(milliseconds to wait=u32 50) -> ()  [unwired: 1 out]
              }
              frame #25 {
                n3847 = local read "EVENT LOG"() -> (w4942:string)
                n3848 = local read "Set Rh"() -> (w4937:dbl)
                n3849 = Number To Fractional String(number=w4937, precision (6)=i16 2) -> (F-format string=w4938:string)  [unwired: 2 in]
                n3850 = Concatenate Strings("Set Humidity [%RH] :" ("Content"), w4938) -> (w4940:string)
                n3851 = call "Event Log.vi"("Content"=w4940, "EVENT LOG"=w4942) -> ("EVENT LOG"=w4941:string)  [unwired: 8 in, 1 out]
                n3852 = local write "EVENT LOG"(w4941) -> ()
              }
              frame #26 {
                n3853 = Wait (ms)(milliseconds to wait=u32 50) -> ()  [unwired: 1 out]
              }
              frame #27 {
                n3854 = local read "EVENT LOG"() -> (w4950:string)
                n3855 = local read "test time"() -> (w4945:dbl)
                n3856 = Number To Fractional String(number=w4945, precision (6)=i16 1) -> (F-format string=w4946:string)  [unwired: 2 in]
                n3857 = Concatenate Strings("Test Duration [mins] :" ("Content"), w4946) -> (w4948:string)
                n3858 = call "Event Log.vi"("Content"=w4948, "EVENT LOG"=w4950) -> ("EVENT LOG"=w4949:string)  [unwired: 8 in, 1 out]
                n3859 = local write "EVENT LOG"(w4949) -> ()
              }
              frame #28 {
                w4951 = dbl[] [] ("History Data")
                w4952 = cluster{"y":dbl, dbl, "y":dbl}[] [] ("History Data")
                w4953 = FALSE ("Visible")
                n3860 = property on="Stroke ( mm )" class="WFChart (strict)"("History Data"=w4952) -> ()  [unwired: 2 in, 2 out]
                n3861 = property on="Stroke ( mm )" class="WFChart (strict)"("History Data"=w4952) -> ()  [unwired: 2 in, 2 out]
                n3862 = property on="Password 3" class="Clust (strict)"("Visible"=w4953) -> ()  [unwired: 2 in, 2 out]
                n3863 = property on="Service Password Log" class="Str"("Visible"=w4953) -> ()  [unwired: 2 in, 2 out]
                n3864 = property on="Electrical Contact Resistance ( % )" class="WFChart (strict)"("History Data"=w4951) -> ()  [unwired: 2 in, 2 out]
                n3865 = property on="Electrical Contact Resistance ( % )" class="WFChart (strict)"("History Data"=w4951) -> ()  [unwired: 2 in, 2 out]
                n3866 = property on="Frictional Force ( N )" class="WFChart (strict)"("History Data"=w4951) -> ()  [unwired: 2 in, 2 out]
                n3867 = property on="Frictional Force ( N )" class="WFChart (strict)"("History Data"=w4951) -> ()  [unwired: 2 in, 2 out]
                n3868 = property on="Temperature ( Deg C )" class="WFChart (strict)"("History Data"=w4951) -> ()  [unwired: 2 in, 2 out]
                n3869 = property on="Temperature ( Deg C )" class="WFChart (strict)"("History Data"=w4951) -> ()  [unwired: 2 in, 2 out]
                n3870 = property on="Coefficient of Friction" class="WFChart (strict)"("History Data"=w4951) -> ()  [unwired: 2 in, 2 out]
                n3871 = property on="Coefficient of Friction" class="WFChart (strict)"("History Data"=w4951) -> ()  [unwired: 2 in, 2 out]
              }
            }
          }
          frame #1 {
            n3872 = stacked-sequence {
              tunnel: 0.0 -> [_ w4972]
              tunnel: [_ w4973] -> _
              frame #0 {
                w4963 = TRUE ("PAUSE")
                n3873 = local read "TOTAL DURATION (SEC)"() -> (w4962:dbl)
                n3874 = property on="Auto Start Test" class="Bool (strict)"("Value"=TRUE ("Auto Start Test")) -> (error out=w4968:errorcluster)  [unwired: 2 in, 1 out]
                n3875 = property on="RUN" class="Bool (strict)"("Visible"=FALSE) -> (error out=w4970:errorcluster)  [unwired: 2 in, 1 out]
                n3876 = call "ELAPSED TIMER VI - demo.vi"("TARGET"=w4962, "RESET"=w4963, "PAUSE"=w4963) -> ()  [unwired: 6 in, 3 out]
                n3877 = Merge Errors(w4968, w4970) -> (w4969:errorcluster)
                n3878 = property on="Heater Button" class="Bool (strict)"(error in=w4969, "Value"=TRUE ("Heater Button")) -> (error out=w4971:errorcluster)  [unwired: 1 in, 1 out]
                n3879 = property on="Humidity" class="Bool (strict)"(error in=w4971, "Value"=TRUE ("Humidity")) -> ()  [unwired: 1 in, 2 out]
                n3880 = property on="Set Frequency:" class="DigNum (strict)"("Value"=50.0 ("Set Frequency:")) -> ()  [unwired: 2 in, 2 out]
                n3881 = property on="Set Stroke:" class="DigNum (strict)"("Value"=1.0 ("Set Stroke:")) -> ()  [unwired: 2 in, 2 out]
                n3882 = property on="Set Temperature:" class="DigNum (strict)"("Value"=60.0 ("Set Temperature:")) -> ()  [unwired: 2 in, 2 out]
                n3883 = property on="Set Humidity:" class="DigNum (strict)"("Value"=53.0 ("Set Humidity:")) -> ()  [unwired: 2 in, 2 out]
                n3884 = local read "EVENT LOG"() -> (w4957:string)
                n3885 = call "Event Log.vi"("Content"="Test Started", "EVENT LOG"=w4957) -> ("EVENT LOG"=w4956:string)  [unwired: 8 in, 1 out]
                n3886 = local write "EVENT LOG"(w4956) -> ()
              }
              frame #1 {
                n3887 = while {
                  shift-right: [w5017] -> w4973
                  shift-left: w4972 -> [w5018]
                  shift-right: [w5006] -> _
                  shift-left: w4972 -> [w5015]
                  shift-right: [w5005] -> _
                  shift-left: w4972 -> [w5013]
                  shift-right: [w5004] -> _
                  shift-left: w4972 -> [w5011]
                  shift-right: [w5002] -> _
                  shift-left: w4972 -> [w5009]
                  shift-right: [w5000] -> _
                  shift-left: w4972 -> [w5007]
                  stop <- w4983 stop-if-true
                  w4985 = FALSE ("PAUSE")
                  w5001 = 0.0  # max
                  # "ff"
                  # "STROKE"
                  # "FREQUENCY"
                  # "HUMIDITY"
                  # "AIR TEMPERATURE"
                  # "SAMPLE TEMPERATURE"
                  n3888 = call "ELAPSED TIMER VI - demo.vi"("TARGET"="TOTAL DURATION (SEC)", "RESET"=w4985, "PAUSE"=w4985) -> ("ELAPSED INDICATION"=w4981:bool, "ELAPSED TIMER"=w4979:dbl)  [unwired: 6 in, 1 out]
                  n3889 = Subtract(x="TOTAL DURATION (SEC)", y=w4979) -> (x-y=w4980:dbl)
                  n3890 = Divide(x=w4979, y="TOTAL DURATION (SEC)") -> (x/y=w4977:dbl)
                  n3891 = Multiply(x=w4977, y=100.0) -> (x*y=w4975:dbl)
                  n3892 = property on="Time Remaining" class="DigNum (strict)"("Value"=w4980) -> ()  [unwired: 2 in, 2 out]
                  n3893 = call "DATA SIMULATION.vi"("Smoothness"=0.03, "PrevVal"=w5018, "MAX"="SAMPLE TEMPERATURE MAX", "MIN"="SAMPLE TEMPERATURE MIN") -> ("Value"=w5017:dbl)  [unwired: 6 in, 1 out]
                  n3894 = call "DATA SIMULATION.vi"("Smoothness"=0.03, "PrevVal"=w5015, "MAX"="AIR TEMPERATURE MAX", "MIN"="AIR TEMPERATURE MIN") -> ("Value"=w5006:dbl)  [unwired: 6 in, 1 out]
                  n3895 = call "DATA SIMULATION.vi"("Smoothness"=0.03, "PrevVal"=w5013, "MAX"="HUMIDITY MAX", "MIN"="HUMIDITY MIN") -> ("Value"=w5005:dbl)  [unwired: 6 in, 1 out]
                  n3896 = call "DATA SIMULATION.vi"("Smoothness"=0.03, "PrevVal"=w5011, "MAX"="FREQUENCY MAX", "MIN"="FREQUENCY MIN") -> ("Value"=w5004:dbl)  [unwired: 6 in, 1 out]
                  n3897 = call "DATA SIMULATION.vi"("Smoothness"=0.01, "PrevVal"=w5009, "MAX"="STROKE MAX", "MIN"="STROKE MIN") -> ("Value"=w5002:dbl)  [unwired: 6 in, 1 out]
                  n3898 = property on="Test Duration Status" class="Slide (strict)"("Value"=w4975) -> ()  [unwired: 2 in, 2 out]
                  n3899 = call "DATA SIMULATION.vi"("Smoothness"=0.1, "PrevVal"=w5007, "MAX"="FF MAX", "MIN"="FF MIN") -> ("Value"=w5000:dbl)  [unwired: 6 in, 1 out]
                  n3900 = Divide(x=w5000, y=1.96) -> (x/y=w4999:dbl)
                  n3901 = property on="TEMP" class="DigNum (strict)"("Value"=w5017) -> ()  [unwired: 2 in, 2 out]
                  n3902 = property on="AIR TEMP" class="DigNum (strict)"("Value"=w5006) -> ()  [unwired: 2 in, 2 out]
                  n3903 = property on="Humidity ( %RH )" class="DigNum (strict)"("Value"=w5005) -> ()  [unwired: 2 in, 2 out]
                  n3904 = property on="Frequency ( Hz )" class="DigNum (strict)"("Value"=w5004) -> ()  [unwired: 2 in, 2 out]
                  n3905 = property on="measured_stroke" class="DigNum (strict)"("Value"=w5002) -> ()  [unwired: 2 in, 2 out]
                  n3906 = property on="FF 3" class="DigNum (strict)"("Value"=w5000) -> ()  [unwired: 2 in, 2 out]
                  n3907 = property on="COF 3" class="DigNum (strict)"("Value"=w4999) -> ()  [unwired: 2 in, 2 out]
                  n3908 = property on="Temperature ( Deg C )" class="WFChart (strict)"("Value"=w5017) -> ()  [unwired: 2 in, 2 out]
                  n3909 = property on="Frictional Force ( N )" class="WFChart (strict)"("Value"=w5000) -> ()  [unwired: 2 in, 2 out]
                  n3910 = property on="Coefficient of Friction" class="WFChart (strict)"("Value"=w4999) -> ()  [unwired: 2 in, 2 out]
                  n3911 = property on="Coefficient of Friction" class="WFChart (strict)"("Value"=w4999) -> ()  [unwired: 2 in, 2 out]
                  n3912 = Bundle("max"=w5001, "Value"=w5002, "max"=w5001) -> (w4998:cluster{"max":dbl, "Value":dbl, "max":dbl})  [unwired: 1 in]
                  n3913 = property on="Stroke ( mm )" class="WFChart (strict)"("Value"=w4998) -> ()  [unwired: 2 in, 2 out]
                  n3914 = property on="Temperature ( Deg C )" class="WFChart (strict)"("Value"=w5017) -> ()  [unwired: 2 in, 2 out]
                  n3915 = property on="Frictional Force ( N )" class="WFChart (strict)"("Value"=w5000) -> ()  [unwired: 2 in, 2 out]
                  n3916 = property on="Stroke ( mm )" class="WFChart (strict)"("Value"=w4998) -> ()  [unwired: 2 in, 2 out]
                  n3917 = Wait (ms)(milliseconds to wait=u32 100) -> ()  [unwired: 1 out]
                  n3918 = property on="DEMO" class="Bool (strict)"() -> ("Value"=w4984:bool)  [unwired: 2 in, 2 out]
